vi "EndTestSuite_WithFailureAtDifferentSubtree_FailedIconSet.vi"() -> (0 "error out":errorcluster)   [LabVIEW 2017, in "ResultTreeListener.Tests.lvlib"]
uses:
  ResultTreeListener.Tests.lvlib
  ResultTree/Icon.ctl
  275d98eb-69a7-4435-8809-2af3ffd1cf1d.vi
  Support/FakeTestSuite/FakeTestSuite.lvclass
  C:/Users/de200256/Code/logmanoriginal/lvunit/TestSuite/TestSuite.lvclass
  Support/FakeTestCase/FakeTestCase.lvclass
  C:/Users/de200256/Code/logmanoriginal/lvunit/Test/Test.lvclass
  Constraint/IsEqual/Create.vi
  ResultTreeListener/ResultTreeListener.lvclass
  Constraint/IsEqual/IsEqual.lvclass
  ResultTree/ResultTree.lvclass
panel:
  in  "Tree":string(tree)
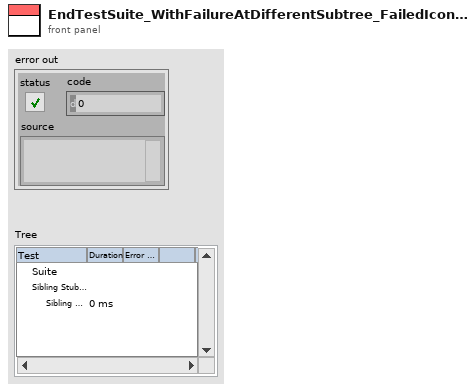
[diagram p1: front panel]
types:
  T1 = typedef "ResultTree.lvclass/Icon.ctl" = enum16{"None", "Passed", "Failed", "Error"}
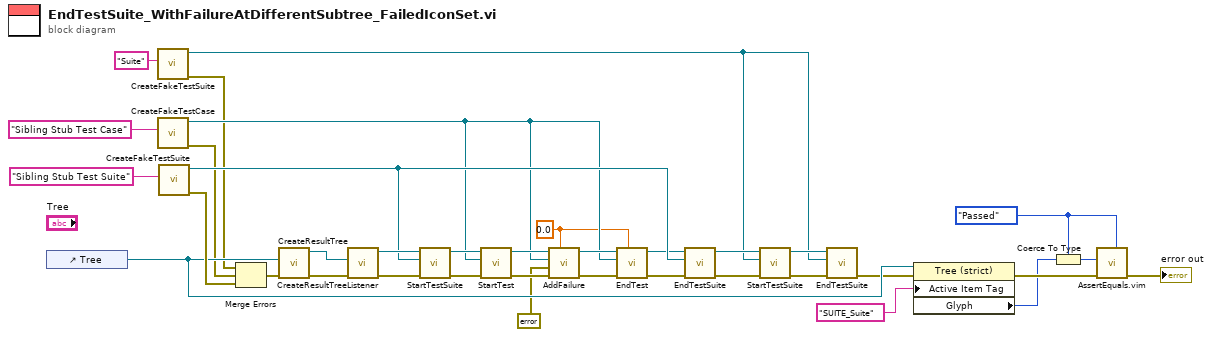
[diagram p0: block diagram]
diagram:
  w9 = 0.0 ("Time")
  w22 = Icon."Passed" ("Active Cell:String")
  n1 = control-ref of="Tree"() -> (w26:refnum<vi>)
  n2 = call "CreateFakeTestSuite.vi"("Name"="Suite") -> ("error out"=w7:errorcluster, "FakeTestSuite out"=w2:refnum<class "FakeTestSuite.lvclass">)  [unwired: 9 in]
  n3 = call "CreateFakeTestCase.vi"("Name"="Sibling Stub Test Case") -> ("error out"=w20:errorcluster, "FakeTestCase out"=w10:refnum<class "FakeTestCase.lvclass">)  [unwired: 9 in]
  n4 = call "CreateFakeTestSuite.vi"("Name"="Sibling Stub Test Suite") -> ("error out"=w29:errorcluster, "FakeTestSuite out"=w28:refnum<class "FakeTestSuite.lvclass">)  [unwired: 9 in]
  n5 = Merge Errors(w7, w20, w29) -> (w21:errorcluster)
  n6 = call "CreateResultTree.vi"("error in (no error)"=w21, "Tree Refnum"=w26) -> ("error out"=w36:errorcluster, "ResultTree out"=w35:refnum<class "ResultTree.lvclass">)  [unwired: 8 in]
  n7 = call "CreateResultTreeListener.vi"("error in (no error)"=w36, "ResultTree"=w35) -> ("error out"=w34:errorcluster, "ResultTreeListener out"=w32:refnum<class "ResultTreeListener.lvclass">)  [unwired: 8 in]
  n8 = call-dynamic "StartTestSuite.vi"("error in (no error)"=w34, "TestSuite"=w28, "ResultTreeListener in"=w32) -> ("error out"=w30:errorcluster, "ResultTreeListener out"=w18:refnum<class "ResultTreeListener.lvclass">)  [unwired: 7 in]
  n9 = call-dynamic "StartTest.vi"("error in (no error)"=w30, "Test"=w10, "ResultTreeListener in"=w18) -> ("error out"=w16:errorcluster, "ResultTreeListener out"=w15:refnum<class "ResultTreeListener.lvclass">)  [unwired: 7 in]
  n10 = call-dynamic "AddFailure.vi"("Time"=w9, "error in (no error)"=w16, "Failure"=errorcluster {"status"=TRUE, "code"=1, "source"="Error."}, "Test"=w10, "ResultTreeListener in"=w15) -> ("error out"=w17:errorcluster, "ResultTreeListener out"=w12:refnum<class "ResultTreeListener.lvclass">)  [unwired: 5 in]
  n11 = call-dynamic "EndTest.vi"("Time"=w9, "error in (no error)"=w17, "Test"=w10, "ResultTreeListener in"=w12) -> ("error out"=w13:errorcluster, "ResultTreeListener out"=w11:refnum<class "ResultTreeListener.lvclass">)  [unwired: 6 in]
  n12 = call-dynamic "EndTestSuite.vi"("error in (no error)"=w13, "TestSuite"=w28, "ResultTreeListener in"=w11) -> ("error out"=w6:errorcluster, "ResultTreeListener out"=w5:refnum<class "ResultTreeListener.lvclass">)  [unwired: 7 in]
  n13 = call-dynamic "StartTestSuite.vi"("error in (no error)"=w6, "TestSuite"=w2, "ResultTreeListener in"=w5) -> ("error out"=w4:errorcluster, "ResultTreeListener out"=w3:refnum<class "ResultTreeListener.lvclass">)  [unwired: 7 in]
  n14 = call-dynamic "EndTestSuite.vi"("error in (no error)"=w4, "TestSuite"=w2, "ResultTreeListener in"=w3) -> ("error out"=w1:errorcluster)  [unwired: 7 in, 1 out]
  n15 = property class="Tree (strict)"(reference=w26, error in=w1, "Active Item Tag"="SUITE_Suite" ("Active Item:Tag")) -> (error out=w27:errorcluster, "Glyph"=w24:i32)  [unwired: 1 out]
  n16 = Coerce To Type(0:w24, 1:w22) -> (2:w23:T1)
  n17 = call "AssertEquals.vim"("Expected"=w22, "error in (no error)"=w27, "Actual"=w23) -> ("error out"=→"error out":errorcluster)  [unwired: 8 in]
